vi "Set Measurement.vi"(6 "Escala":dbl, 8 "error in (no error)":errorcluster, 9 "Range ON/OFF":bool, 10 "Grandeza Elétrica":string, 11 "U1252 in":refnum<class "U1252.lvclass">) -> (0 "error out":errorcluster, 3 "U1252 out":refnum<class "U1252.lvclass">)   [LabVIEW 2015, in "U1252.lvclass"]
uses:
  U1252.lvclass
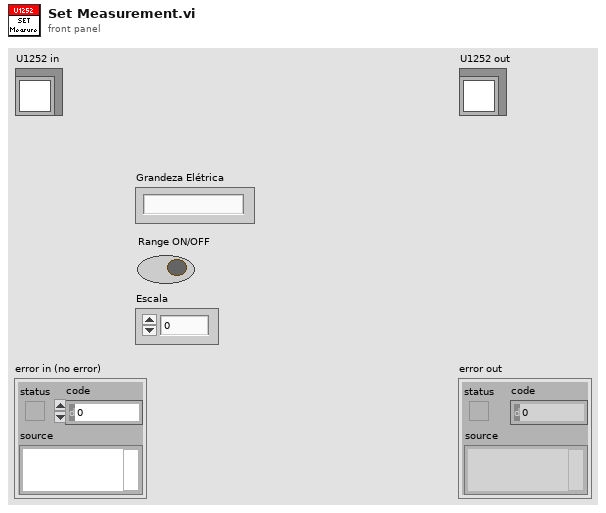
[diagram p1: front panel]
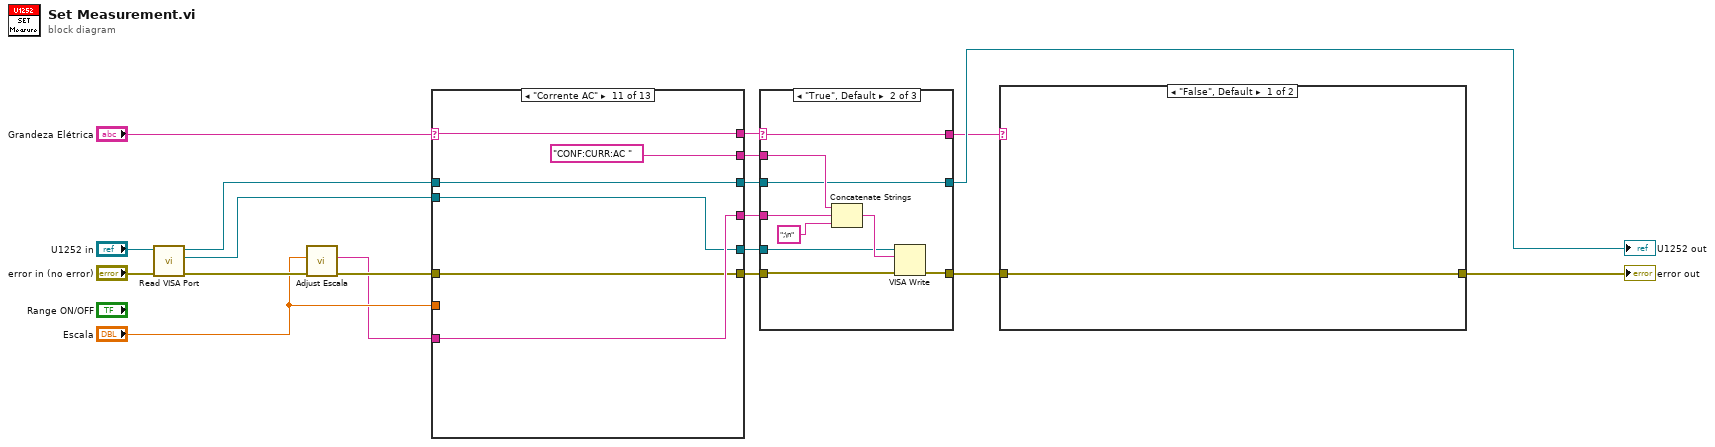
[diagram p0: block diagram]
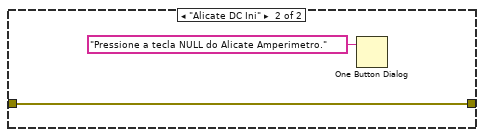
[diagram p2: hidden frame]
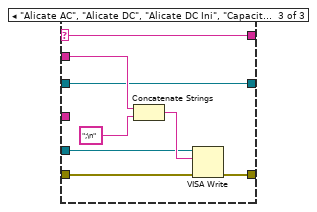
[diagram p4: hidden frame]
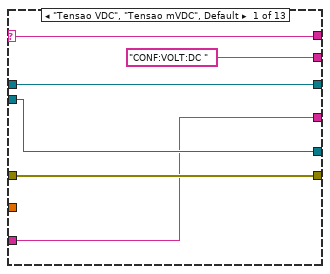
[diagram p5: hidden frame]
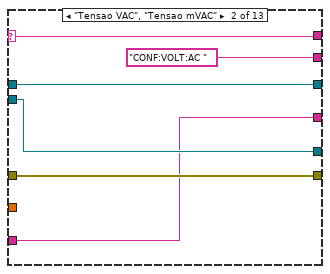
[diagram p6: hidden frame]
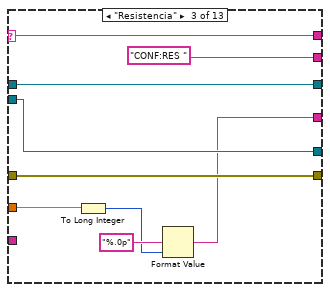
[diagram p7: hidden frame]
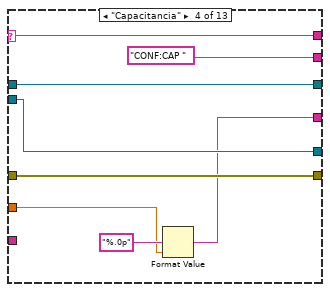
[diagram p8: hidden frame]
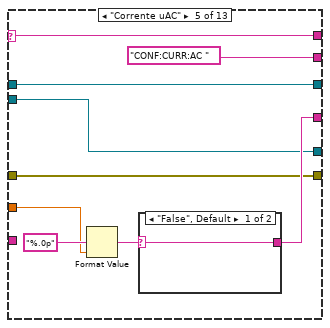
[diagram p9: hidden frame]
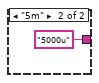
[diagram p10: hidden frame]
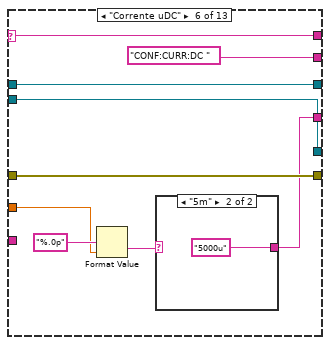
[diagram p11: hidden frame]
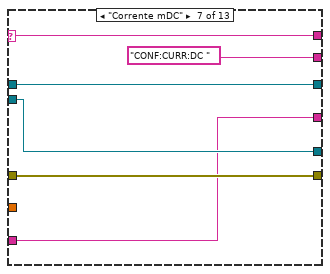
[diagram p13: hidden frame]
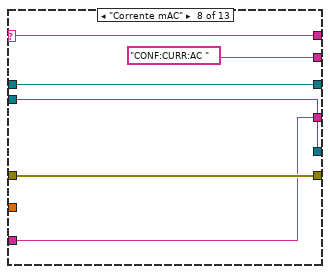
[diagram p14: hidden frame]
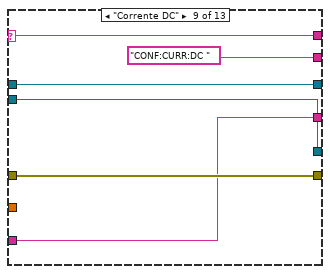
[diagram p15: hidden frame]
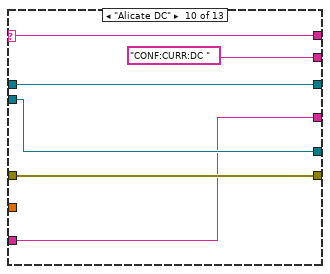
[diagram p16: hidden frame]
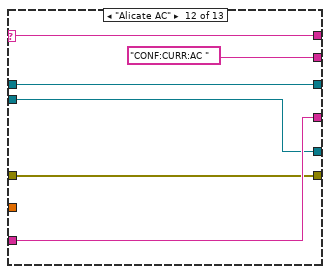
[diagram p17: hidden frame]
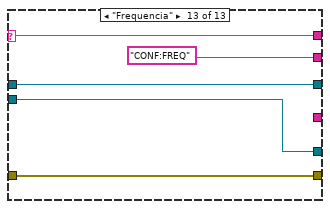
[diagram p18: hidden frame]
diagram:
  n1 = call-dynamic "Read VISA Port.vi"("error in (no error)"="error in (no error)", "Device in"="U1252 in") -> ("error out"=w10:errorcluster, "VISA Port"=w1:refnum<visa-resource-name>, "Device out"=w17:refnum<class "U1252.lvclass">)  [unwired: 7 in]
  n2 = call "Adjust Escala.vi"("error in (no error)"=w10, "Escala"="Escala") -> ("error out"=w11:errorcluster, "Escala String"=w8:string)  [unwired: 8 in]
  n3 = case shown="\"Corrente AC\"" "Grandeza Elétrica" {
    selector: "Grandeza Elétrica" -> [w24 w30 w39 w47 w57 w67 w75 w81 w87 w93 w100 w106 w111]
    tunnel: w11 -> [w22 w28 w37 w45 w51 w65 w73 w79 w85 w91 w96 w102 w108]
    tunnel: w1 -> [w21 w27 w38 w46 w49 w66 w74 w80 w86 w92 w95 w101 w107]
    tunnel: w17 -> [w25 w31 w40 w48 w50 w68 w76 w82 w88 w94 w97 w103 w109]
    tunnel: [w25 w31 w40 w48 w50 w68 w76 w82 w88 w94 w97 w103 w109] -> w6
    tunnel: [w24 w30 w39 w47 w57 w67 w75 w81 w87 w93 w100 w106 w111] -> w7
    tunnel: ["CONF:VOLT:DC " "CONF:VOLT:AC " "CONF:RES " "CONF:CAP " "CONF:CURR:AC " "CONF:CURR:DC " "CONF:CURR:DC " "CONF:CURR:AC " "CONF:CURR:DC " "CONF:CURR:DC " "CONF:CURR:AC " "CONF:CURR:AC " "CONF:FREQ"] -> w15
    tunnel: [w22 w28 w37 w45 w51 w65 w73 w79 w85 w91 w96 w102 w108] -> w14
    tunnel: [w21 w27 w38 w46 w49 w66 w74 w80 w86 w92 w95 w101 w107] -> w13
    tunnel: w8 -> [w20 w26 _ _ _ _ w71 w77 w83 w89 w98 w104 _]
    tunnel: [w20 w26 w32 w41 w52 w60 w71 w77 w83 w89 w98 w104 _] -> w12
    tunnel: "Escala" -> [_ _ w34 w42 w54 w62 _ _ _ _ _ _ _]
    frame "Tensao VDC", "Tensao mVDC", Default {
    }
    frame "Tensao VAC", "Tensao mVAC" {
    }
    frame "Resistencia" {
      n4 = To Long Integer(number=w34) -> (32bit integer=w33:i32)
      n5 = Format Value(format string="%.0p", value (0)=w33) -> (output string=w32:string)  [unwired: 1 in]
    }
    frame "Capacitancia" {
      n6 = Format Value(format string="%.0p", value (0)=w42) -> (output string=w41:string)  [unwired: 1 in]
    }
    frame "Corrente uAC" {
      n7 = Format Value(format string="%.0p", value (0)=w54) -> (output string=w53:string)  [unwired: 1 in]
      n8 = case shown="\"False\", Default" w53 {
        selector: w53 -> [w58 _]
        tunnel: [w58 "5000u"] -> w52
        frame "False", Default {
        }
        frame "5m" {
        }
      }
    }
    frame "Corrente uDC" {
      n9 = Format Value(format string="%.0p", value (0)=w62) -> (output string=w61:string)  [unwired: 1 in]
      n10 = case shown="\"5m\"" w61 {
        selector: w61 -> [w69 _]
        tunnel: [w69 "5000u"] -> w60
        frame "False", Default {
        }
        frame "5m" {
        }
      }
    }
    frame "Corrente mDC" {
    }
    frame "Corrente mAC" {
    }
    frame "Corrente DC" {
    }
    frame "Alicate DC" {
    }
    frame "Corrente AC" {
    }
    frame "Alicate AC" {
    }
    frame "Frequencia" {
    }
  }
  n11 = case shown="\"True\", Default" w7 {
    selector: w7 -> [w112 w119 w124]
    tunnel: w15 -> [_ w122 w130]
    tunnel: w14 -> [w113 w115 w129]
    tunnel: w13 -> [_ w116 w128]
    tunnel: w12 -> [_ w121 _]
    tunnel: [w113 w118 w127] -> w3
    tunnel: [w114 w120 w126] -> w5
    tunnel: w6 -> [w114 w120 w126]
    tunnel: [w112 w119 w124] -> w4
    frame "Resistencia" {
    }
    frame "True", Default {
      n12 = Concatenate Strings(w122, w121, ";\n" ("string")) -> (w117:string)
      n13 = VISA Write(VISA resource name=w116, write buffer=w117, error in (no error)=w115) -> (error out=w118:errorcluster)  [unwired: 2 out]
    }
    frame "Alicate AC", "Alicate DC", "Alicate DC Ini", "Capacitancia" {
      n14 = Concatenate Strings(w130, ";\n" ("string")) -> (w131:string)
      n15 = VISA Write(VISA resource name=w128, write buffer=w131, error in (no error)=w129) -> (error out=w127:errorcluster)  [unwired: 2 out]
    }
  }
  "U1252 out" <- w5
  n16 = case shown="\"False\", Default" w4 {
    tunnel: w3 -> [w132 w134]
    tunnel: [w132 w134] -> w2
    frame "False", Default {
    }
    frame "Alicate DC Ini" {
      n17 = One Button Dialog(message="Pressione a tecla NULL do Alicate Amperimetro.") -> ()  [unwired: 1 in, 1 out]
    }
  }
  "error out" <- w2
